vi "Into.vi"(0 "Pair":refnum<class "Pair.lvclass">) -> (1 "Key":string, 2 "Value":refnum<class "Datum.lvclass">)   [LabVIEW 2018, in "Toolkit.lvlib" / "Data.lvlib" / "Pair.lvclass"]
doc: "Breaks the Pair object into its key and value components"
uses:
  Pair.lvclass
  Datum/Datum.lvclass
  Pair.lvclass/Pair.ctl
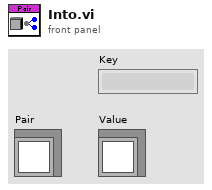
[diagram p1: front panel]
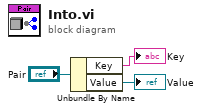
[diagram p0: block diagram]
diagram:
  n1 = Unbundle By Name("Pair") -> ("Key"=→"Key":string, "Value"=→"Value":refnum<class "Datum.lvclass">)
